vi "ImageRotator.vi"() -> ()   [LabVIEW 2018]
uses:
  ImageRotator.dll
panel:
  out "2D Picture":picture
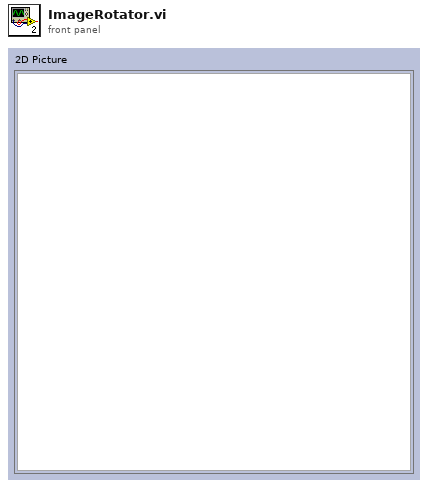
[diagram p1: front panel]
types:
  T1 = typedef "imagedata.ctl" = cluster{"image type":i32, "image depth":i32, "image":u8[], "mask":u8[], "colors":u32[], "Rectangle":cluster{"left":i16, "top":i16, "right":i16, "bottom":i16}}
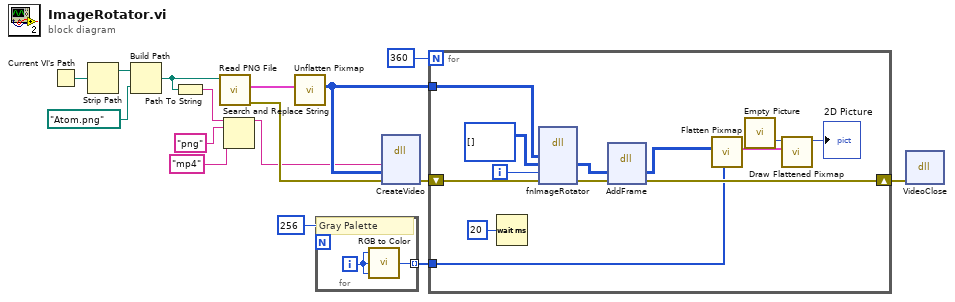
[diagram p0: block diagram]
diagram:
  n1 = Current VI's Path() -> (path=w8:path)
  n2 = Strip Path(path=w8) -> (stripped path=w6:path)  [unwired: 1 out]
  n3 = Build Path(base path=w6, name or relative path=path "Atom.png") -> (appended path=w5:path)
  n4 = Path To String(path=w5) -> (string=w4:string)
  n5 = call <vilib>:"Read PNG File.vi"("path to PNG file"=w5) -> ("error out"=w13:errorcluster, "image data"=w15:T1)  [unwired: 8 in, 1 out]
  n6 = Search and Replace String(input string=w4, search string="png", replace string="mp4" ("replace string (\"\")")) -> (result string=w1:string)  [unwired: 5 in, 3 out]
  n7 = call <vilib>:"Unflatten Pixmap.vi"("image data"=w15) -> ("8-bit pixmap"=w14:u8[][])  [unwired: 4 in, 6 out]
  n8 = for {
    N: 256 -> [_]
    tunnel: [w17] -> w9 mode=indexing
    i -> [w18]
    # "Gray Palette"
    n9 = call <vilib>:"RGB to Color.vi"("B"=w18, "G"=w18, "R"=w18) -> ("Color"=w17:u32)
  }
  n10 = dll-call lib="D:/MATLAB Test/ImageRotator/ImageRotator/ImageRotator.dll" fn="CreateVideo"("file"=w1, "image"=w14, "error"=w13) -> ("error"=w12:errorcluster)  [unwired: 6 in, 2 out]
  n11 = for {
    N: 360 -> [_]
    tunnel: w14 -> [w26]
    tunnel: w9 -> [w22]
    shift-right: [w23] -> w11
    shift-left: w12 -> [w20]
    i -> [w21]
    n12 = Wait (ms)(milliseconds to wait=u32 20) -> ()  [unwired: 1 out]
    n13 = dll-call lib="D:/MATLAB Test/ImageRotator/ImageRotator/ImageRotator.dll" fn="fnImageRotator"("src"=w26, "dst"=u8[][] [] ("8-bit pixmap"), "angle"=w21, w20) -> ("dst"=w25:u8[][], w24:errorcluster)  [unwired: 6 in, 2 out]
    n14 = dll-call lib="D:/MATLAB Test/ImageRotator/ImageRotator/ImageRotator.dll" fn="AddFrame"("image"=w25, "error"=w24) -> ("image"=w19:u8[][], "error"=w23:errorcluster)  [unwired: 4 in, 2 out]
    n15 = call <vilib>:"Flatten Pixmap.vi"("colors"=w22, "8-bit pixmap"=w19) -> ("image data"=w28:T1)  [unwired: 9 in]
    n16 = call "Empty Picture"() -> ("empty picture"=w29:picture)
    n17 = call <vilib>:"Draw Flattened Pixmap.vi"("image data"=w28, "picture"=w29) -> ("new picture"=→"2D Picture":picture)  [unwired: 7 in]
  }
  n18 = dll-call lib="D:/MATLAB Test/ImageRotator/ImageRotator/ImageRotator.dll" fn="VideoClose"("error"=w11) -> ()  [unwired: 5 in, 2 out]
